vi "WriteADCToSetUp.vi"(1 "adc_res(dig)":i32, 2 "ASCIISetUp":string) -> (6 "ASCIISetUpOut":string)   [LabVIEW 2017]
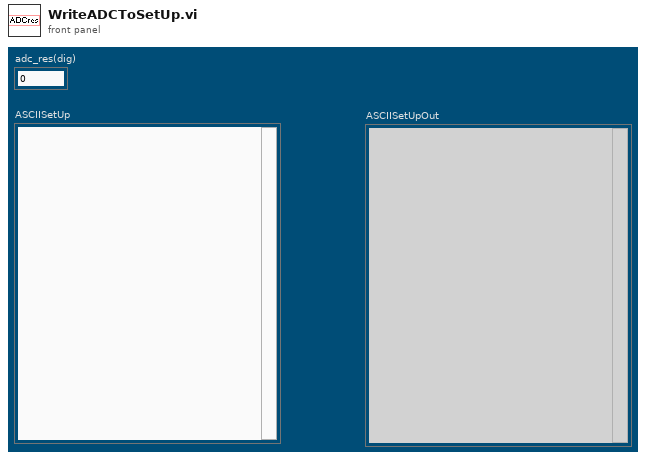
[diagram p1: front panel]
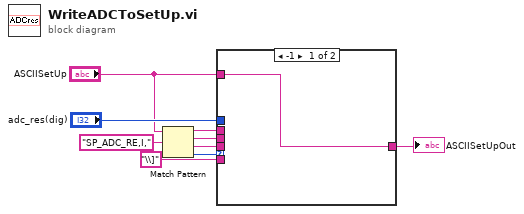
[diagram p0: block diagram]
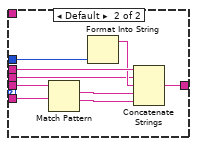
[diagram p2: hidden frame]
diagram:
  n1 = Match Pattern(string="ASCIISetUp", regular expression="SP_ADC_RE,I,") -> (before substring=w7:string, match substring=w6:string, after substring=w4:string, offset past match=w2:i32)  [unwired: 1 in]
  n2 = case shown="-1" w2 {
    tunnel: [w10 w19] -> w9
    tunnel: "adc_res(dig)" -> [_ w18]
    tunnel: w7 -> [_ w15]
    tunnel: w6 -> [_ w13]
    tunnel: "\\]" ("regular expression") -> [_ w12]
    tunnel: w4 -> [_ w11]
    tunnel: "ASCIISetUp" -> [w10 _]
    frame -1 {
    }
    frame Default {
      n3 = Match Pattern(string=w11, regular expression=w12) -> (match substring=w16:string, after substring=w17:string)  [unwired: 1 in, 2 out]
      n4 = Format Into String(w18) -> (resulting string=w14:string)  [unwired: 3 in, 1 out]
      n5 = Concatenate Strings(w15, w13, w14, w16, w17) -> (w19:string)
    }
  }
  "ASCIISetUpOut" <- w9
